vi "Solvent Data Extractor.vi"(8 "Error In":errorcluster, 9 "Solvent Data":variant[][](array[variant])=[[variant]], 10 "Solvent Name":string) -> (0 "Error Out":errorcluster, 2 "Exists?":bool, 3 "Solvent Information":cluster{"Solvent Name":string, "Solvent ID":i32})   [LabVIEW 2020]
uses:
  <vilib>/addons/database/_DB Variant To Data/Database Variant To Data.xnode
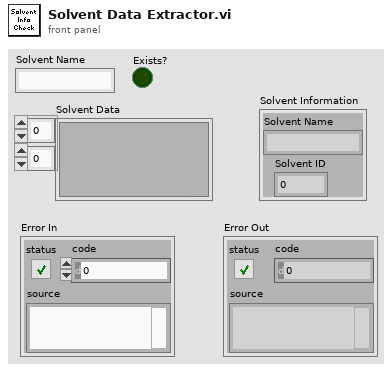
[diagram p1: front panel]
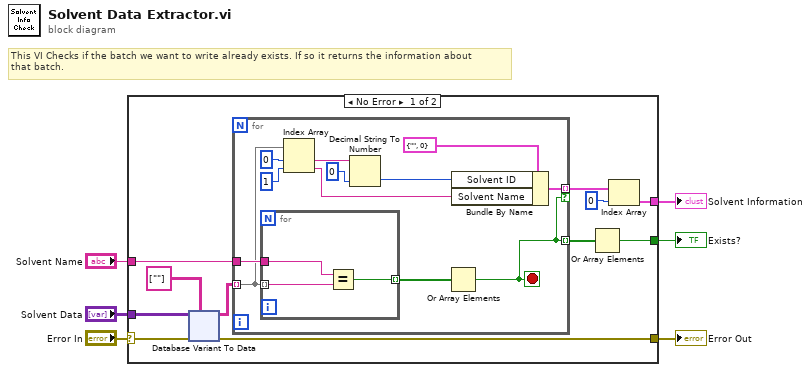
[diagram p0: block diagram]
diagram:
  # "This VI Checks if the batch we want to write already exists. If so it returns the information about\nthat batch."
  n1 = case shown="No Error" "Error In" {
    selector: "Error In" -> [w13 w77]
    tunnel: "Solvent Data" -> [w14 _]
    tunnel: "Solvent Name" -> [w12 _]
    tunnel: [w10 _] -> w3
    tunnel: [w11 w77] -> w2
    tunnel: [w7 _] -> w1
    frame No Error {
      n2 = xnode "Database Variant To Data"("database variant"=w14, "error in (no error)"=w13, "type"=string[][] [[""]] ("columns")) -> ("data"=w15:string[][], "error out"=w11:errorcluster)
      n3 = for {
        tunnel: w15 -> [w19] mode=indexing
        tunnel: w12 -> [w29]
        tunnel: [w18] -> w16 mode=indexing
        tunnel: [w20] -> w9 mode=indexing if=w18
        stop <- w18 stop-if-true
        n4 = for {
          tunnel: w19 -> [w31] mode=indexing
          tunnel: w29 -> [w32]
          tunnel: [w30] -> w28 mode=indexing
          n5 = Equal?(x=w32, y=w31) -> (x = y?=w30:bool)
        }
        n6 = Index Array(array=w19, index #1=0 ("index"), index #2=1 ("index")) -> (element #1=w25:string, element #2=w22:string)
        n7 = Decimal String To Number(string=w25, default (0L)=0 ("default (0 I32)")) -> (number=w21:i32)  [unwired: 1 in, 1 out]
        n8 = Or Array Elements(Boolean array=w28) -> (logical OR=w18:bool)
        n9 = Bundle By Name(cluster=cluster{"Solvent Name":string, "Solvent ID":i32} {"Solvent Name"="", "Solvent ID"=0} ("output cluster"), "Solvent ID"=w21, "Solvent Name"=w22) -> (w20:cluster{"Solvent Name":string, "Solvent ID":i32})
      }
      n10 = Or Array Elements(Boolean array=w16) -> (logical OR=w10:bool)
      n11 = Index Array(array=w9, index=0) -> (element=w7:cluster{"Solvent Name":string, "Solvent ID":i32})
    }
    frame Error {
    }
  }
  "Exists?" <- w3
  "Error Out" <- w2
  "Solvent Information" <- w1
